vi "Pre Launch Init.vi"(11 "Subpanel Inserter in":refnum<class "Subpanel Inserter.lvclass">) -> (0 "error out":errorcluster, 3 "Subpanel Inserter out":refnum<class "Subpanel Inserter.lvclass">)   [LabVIEW 2014, in "Subpanel Insertion.lvlib" / "Subpanel Inserter.lvclass"]
doc: "(<B>Filename</B>: Actor Framework.lvlib:Actor.lvclass:Pre Launch Init.vi)\n\nDefines behavior that occurs after the Launch Nested Actor method is invoked but before the actor's Actor Core method begins running.\n\nBy default, this method does nothing. A descendant class may override it to define behavior."
uses:
  Subpanel Inserter.lvclass
  <vilib>/ActorFramework/Actor/Actor.lvclass
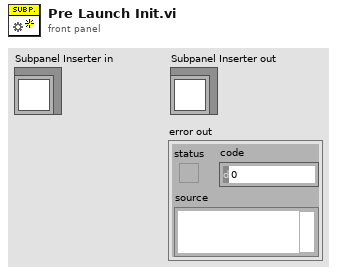
[diagram p1: front panel]
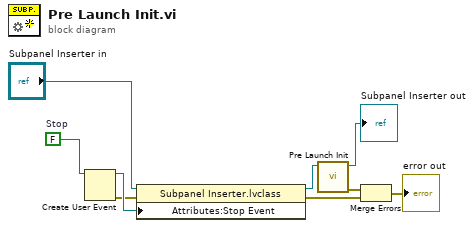
[diagram p0: block diagram]
diagram:
  w6 = FALSE  # Stop
  n1 = Create User Event(user event datatype=w6) -> (user event=w5:refnum<user-event>, error out=w4:errorcluster)  [unwired: 1 in]
  n2 = property class="Subpanel Inserter.lvclass"(reference="Subpanel Inserter in", error in=w4, "Attributes:Stop Event"=w5) -> (reference out=w7:refnum<class "Subpanel Inserter.lvclass">, error out=w1:errorcluster)
  n3 = call-parent "Pre Launch Init.vi"("Actor in"=w7) -> ("error out"=w3:errorcluster, "Actor out"=→"Subpanel Inserter out":refnum<class "Subpanel Inserter.lvclass">)  [unwired: 9 in]
  n4 = Merge Errors(w3, w1) -> (→"error out":errorcluster)
